vi "Set XSSFWorkbook.vi"(8 "error in (no error)":errorcluster, 10 "XSSFWorkbook":refnum<k24>, 11 "Excel XML in":refnum<class "Excel XML.lvclass">) -> (0 "error out":errorcluster, 3 "Excel XML out":refnum<class "Excel XML.lvclass">)   [LabVIEW 2013, in "Excel XML.lvclass"]
uses:
  Excel XML.lvclass
  C:/PhaeronGit/LVNPOI/Resources/NPOI 2.1.1 dotnet4/NPOI.OOXML.dll
  Resources/NPOI 2.1.1 dotnet4/NPOI.OOXML.dll
  Excel XML.lvclass/Excel XML.ctl
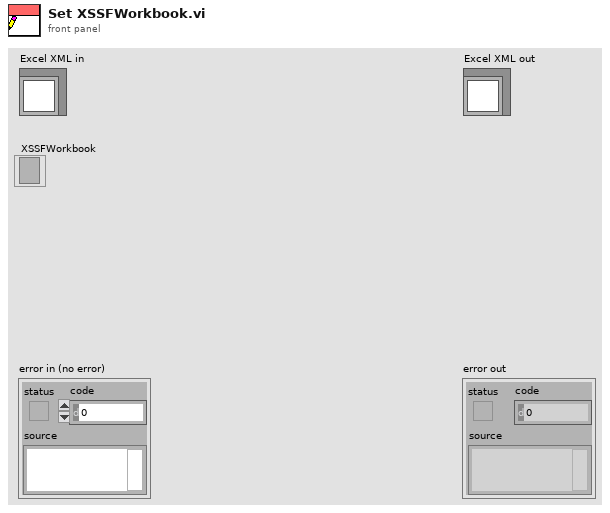
[diagram p1: front panel]
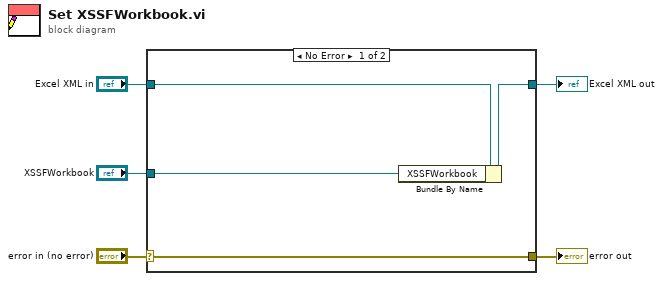
[diagram p0: block diagram]
diagram:
  n1 = case shown="No Error" "error in (no error)" {
    selector: "error in (no error)" -> [w9 w10]
    tunnel: [w9 w10] -> w4
    tunnel: [w7 w11] -> w2
    tunnel: "Excel XML in" -> [w8 w11]
    tunnel: "XSSFWorkbook" -> [w6 _]
    frame No Error {
      n2 = Bundle By Name(cluster=w8, "XSSFWorkbook"=w6) -> (w7:refnum<class "Excel XML.lvclass">)
    }
    frame Error {
    }
  }
  "error out" <- w4
  "Excel XML out" <- w2
